vi "Read Transmission Spectrum without saving.vi"(0 "VISA IN":refnum<visa-resource-name>="COM1" caption="serial number", 5 "error in (no error)":errorcluster caption="错误输入（无错误）") -> (14 "VISA OUT":refnum<visa-resource-name>, 15 "DATA":u8[](array[numeric]) format="%02x", 19 "error out":errorcluster caption="错误输出")   [LabVIEW 2013]
uses:
  <vilib>/Analysis/6fits.llb/General Linear Fit Algorithm.ctl
  <vilib>/Analysis/NI_AALPro.lvlib
panel:
  out "String":string
  out "Best Polynomial Fit":dbl[](array[numeric])
  out "XY Graph Fitting":cluster{i32[], "Best Polynomial Fit":dbl[]}[](graph)
  in  "Analyze length":i32=1000
  in  "Sample Start Index":i32
  out "Error Times":dbl
  out "Numeric":i32
  out "XY Graph":cluster{i32[], u32[]}(graph)
  out "read buffer":string
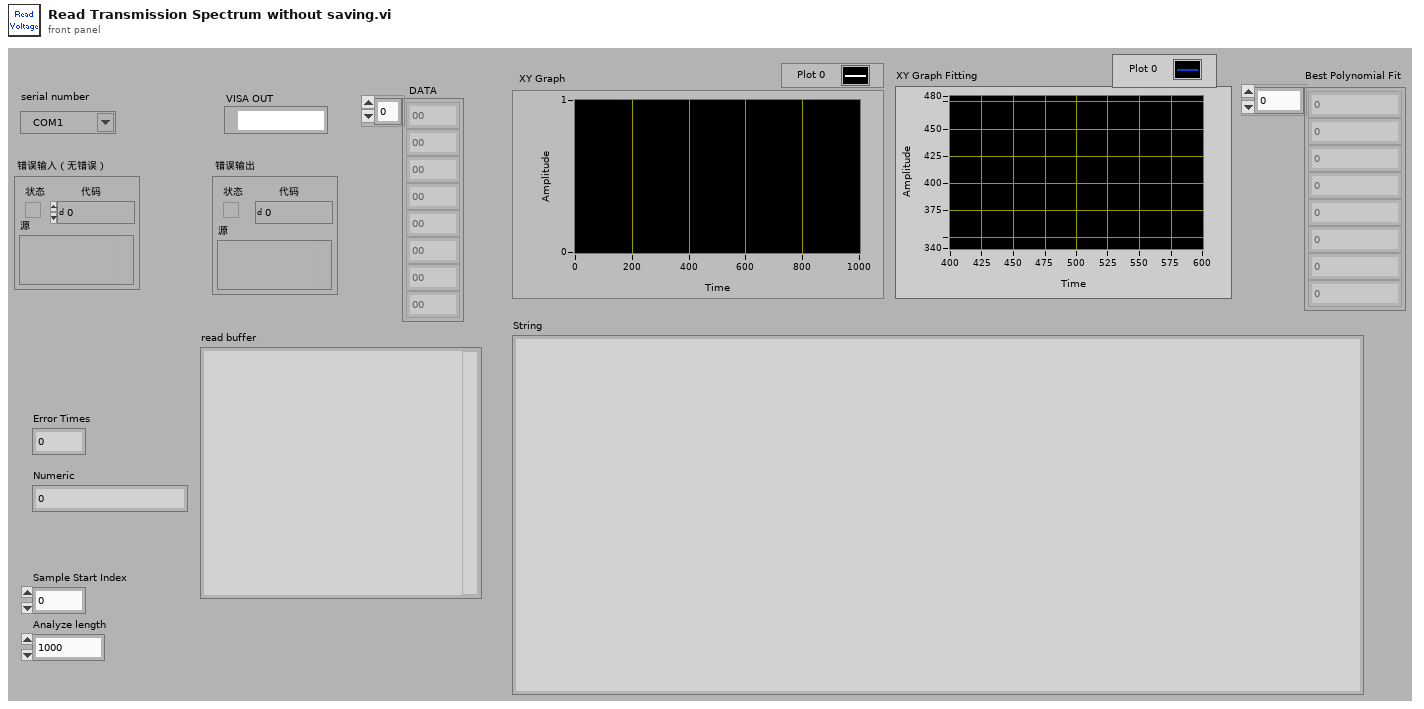
[diagram p1: front panel]
types:
  T1 = typedef "NI_AALPro.lvlib/General Linear Fit Algorithm.ctl" = u16
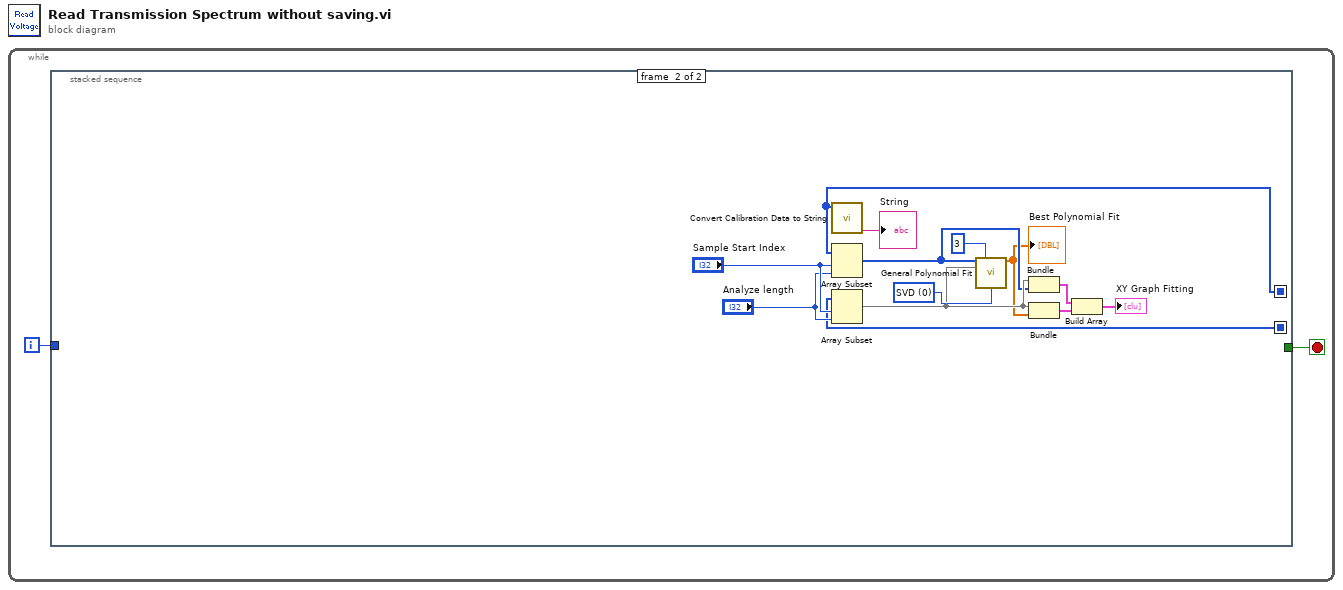
[diagram p0: block diagram]
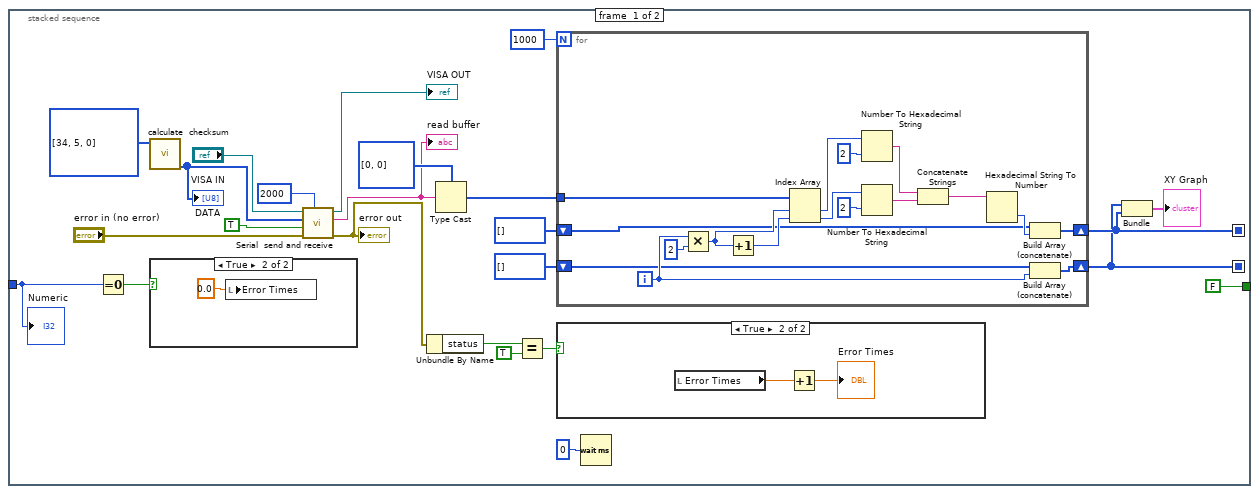
[diagram p2: hidden frame]
diagram:
  n1 = while {
    i -> [w2]
    stop <- w1 stop-if-true
    n2 = stacked-sequence {
      seq-local: [w4 _] -> [_ w48]
      seq-local: [w3 _] -> [_ w47]
      tunnel: w2 -> [w8 _]
      tunnel: [FALSE _] -> w1
      frame #0 {
        n3 = Equal To 0?(x=w8) -> (x = 0?=w7:bool)
        n4 = call "calculate  checksum.vi"("front command"=u8[] [34, 5, 0]) -> ("DATA"=w26:u8[])  [unwired: 9 in, 1 out]
        "DATA" <- w26
        n5 = case shown="True" w7 {
          frame False {
          }
          frame True {
            n6 = local write "Error Times"(0.0 ("Error Times")) -> ()
          }
        }
        n7 = call "Serial  send and receive.vi"("读取字节总数"=u32 2000, "error in (no error)"="error in (no error)", "读取"=TRUE, "command"=w26, "VISA IN"="VISA IN") -> ("error out"=w12:errorcluster, "read buffer"=w14:string, "VISA OUT"=→"VISA OUT":refnum<visa-resource-name>)  [unwired: 2 in, 2 out]
        "error out" <- w12
        "read buffer" <- w14
        n8 = Unbundle By Name(w12) -> ("status"=w11:bool)
        n9 = Type Cast(type=u8[] [0, 0], x=w14) -> (*(type *) &x=w18:u8[])
        n10 = Equal?(x=w11, y=TRUE) -> (x = y?=w9:bool)
        n11 = for {
          N: 1000 -> [_]
          tunnel: w18 -> [w44]
          shift-right: [w35] -> w4
          shift-left: u32[] [] -> [w33]
          shift-right: [w31] -> w3
          shift-left: i32[] [] -> [w30]
          i -> [w32]
          n12 = Multiply(x=w32, y=i16 2 ("宽度(-)")) -> (x*y=w37:i32)
          n13 = Increment(x=w37) -> (x+1=w36:i32)
          n14 = Index Array(array=w44, index #1=w37, index #2=w36) -> (element #1=w46:u8, element #2=w43:u8)
          n15 = Number To Hexadecimal String(1:i16 2 ("宽度(-)"), 2:w46) -> (0:w45:string)
          n16 = Number To Hexadecimal String(1:i16 2 ("宽度(-)"), 2:w43) -> (0:w42:string)
          n17 = Concatenate Strings(w45, w42) -> (w39:string)
          n18 = Hexadecimal String To Number(string=w39) -> (number=w34:u32)  [unwired: 2 in, 1 out]
          n19 = Build Array (concatenate)(w33, w34) -> (w35:u32[])
          n20 = Build Array (concatenate)(w30, w32) -> (w31:i32[])
        }
        n21 = case shown="True" w9 {
          frame False {
          }
          frame True {
            n22 = local read "Error Times"() -> (w28:dbl)
            n23 = Increment(x=w28) -> (x+1=→"Error Times":dbl)
          }
        }
        n24 = Wait (ms)(milliseconds to wait=u32 0) -> ()  [unwired: 1 out]
        n25 = Bundle(w3, w4) -> (→"XY Graph":cluster{i32[], u32[]})  [unwired: 1 in]
        "Numeric" <- w8
      }
      frame #1 {
        w59 = T1 0 items=["SVD", "Givens", "Givens2", "Householder", "LU Decomposition", "Cholesky", "SVD for Rank Deficient H"] ("algorithm")
        n26 = call "Convert Calibration Data to String.vi"("Input"=w48) -> ("String"=→"String":string)  [unwired: 9 in, 1 out]
        n27 = Array Subset(array=w48, index="Sample Start Index", length="Analyze length") -> (w51:u32[])
        n28 = Array Subset(array=w47, index="Sample Start Index", length="Analyze length") -> (w52:i32[])
        n29 = call <vilib>:"General Polynomial Fit.vi"("Y"=w51, "polynomial order"=3, "X"=w52, "algorithm"=w59) -> ("Best Polynomial Fit"=w50:dbl[])  [unwired: 8 in, 3 out]
        "Best Polynomial Fit" <- w50
        n30 = Bundle(w52, w51) -> (w53:cluster{i32[], u32[]})  [unwired: 1 in]
        n31 = Bundle(w52, "Best Polynomial Fit"=w50) -> (w54:cluster{i32[], "Best Polynomial Fit":dbl[]})  [unwired: 1 in]
        n32 = Build Array(w53, w54) -> (→"XY Graph Fitting":cluster{i32[], "Best Polynomial Fit":dbl[]}[])
      }
    }
  }
